vi "testing.vi"   [LabVIEW 2023]
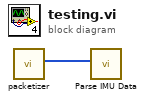
[diagram p0: block diagram]
diagram:
  n1 = call "packetizer.vi"() -> ("Packet Payload"=w1:u8[])  [unwired: 11 in]
  n2 = call "Parse IMU Data.vi"("Packet"=w1) -> ()  [unwired: 11 in]
